vi "设置权限.vi"() -> (7 "Cancelled?":bool caption="取消？", 8 "验证成功":bool, 9 "权限选择 2":u16(ring) caption="确定" items=["Admin", "User"])   [LabVIEW 2017]
doc: "该模板用于创建能够进行事件处理的对话框。"
panel:
  in  "权限选择":u16(ring) caption="确定" items=["Admin", "User"]
  in  "修改密码":bool caption="确定"
  in  "密码":string
  in  "Cancel":bool caption="取消"
  in  "验证":bool caption="确定"
  # "权限验证"
  # "密码"
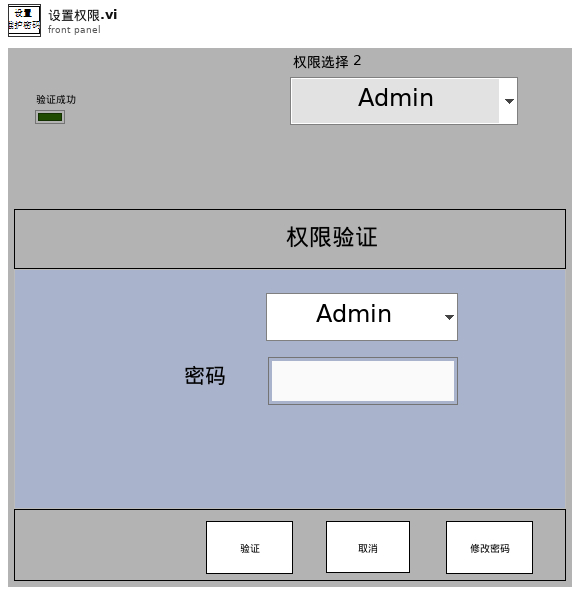
[diagram p1: front panel]
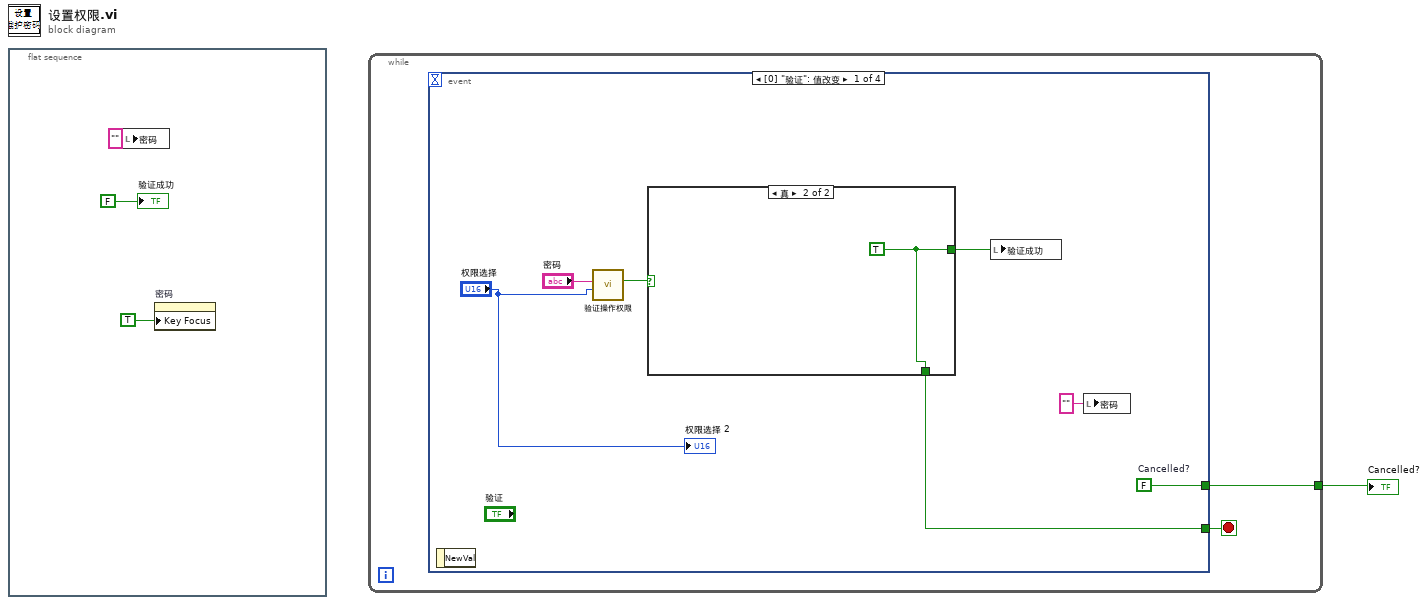
[diagram p0: block diagram]
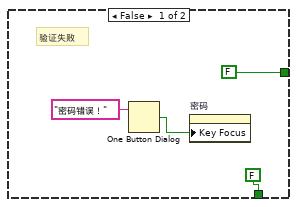
[diagram p2: hidden frame]
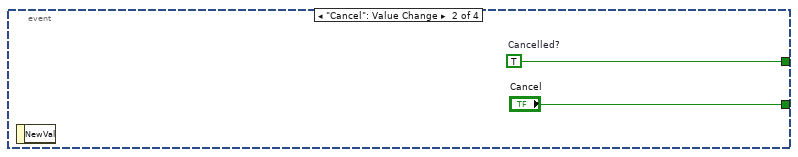
[diagram p3: hidden frame]
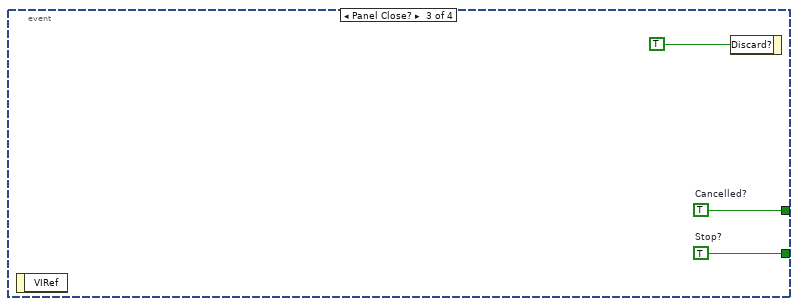
[diagram p4: hidden frame]
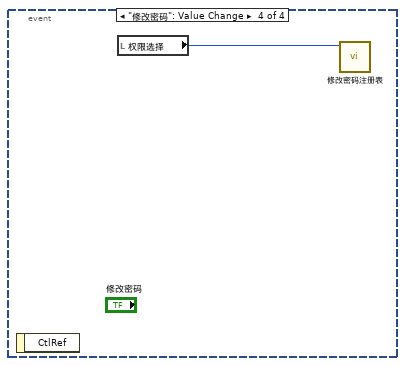
[diagram p5: hidden frame]
diagram:
  n1 = flat-sequence {
    frame #0 {
      n2 = local write "密码"("" ("用户名")) -> ()
      n3 = property on="密码" class="Str"("Key Focus"=TRUE ("键选中")) -> ()  [unwired: 2 in, 2 out]
      "验证成功" <- FALSE ("验证成功")
    }
  }
  n4 = while {
    tunnel: [w5] -> w1
    stop <- w6 stop-if-true
    n5 = event shown="[0] \"验证\": 值改变" {
      selector: _ -> [_ _ _ _]
      dyn-events: _ -> [_ _ _ _]
      timeout: _ -> [_ _ _ _]
      tunnel: [w8 "Cancel" w22 _] -> w6
      tunnel: [w13 w20 w21 _] -> w5
      event "验证": Value Change {
        w13 = FALSE  # Cancelled?
        n6 = event-data() -> ()  [unwired: 1 in, 1 out]
        n7 = call "验证操作权限.vi"("权限选择"="权限选择", "密码"="密码") -> ("验证成功"=w10:bool)  [unwired: 9 in]
        n8 = case shown="真" w10 {
          tunnel: [FALSE ("验证成功") w18] -> w9
          tunnel: [FALSE ("验证成功") w18] -> w8
          frame False {
            # "验证失败"
            n9 = One Button Dialog(message="密码错误！" ("消息")) -> (true=w14:bool)  [unwired: 1 in]
            n10 = property on="密码" class="Str"("Key Focus"=w14) -> ()  [unwired: 2 in, 2 out]
          }
          frame True {
            w18 = TRUE ("验证成功")
          }
        }
        n11 = local write "验证成功"(w9) -> ()
        n12 = local write "密码"("" ("用户名")) -> ()
        "权限选择 2" <- "权限选择"
      }
      event "Cancel": Value Change {
        w20 = TRUE  # Cancelled?
        n13 = event-data() -> ()  [unwired: 1 in, 1 out]
      }
      event Panel Close? {
        w21 = TRUE  # Cancelled?
        w22 = TRUE  # Stop?
        n14 = event-data() -> ()  [unwired: 1 in, 1 out]
        n15 = event-data("Discard?"=TRUE) -> ()  [unwired: 1 in, 1 out]
      }
      event "修改密码": Value Change {
        n16 = event-data() -> ()  [unwired: 1 in, 1 out]
        n17 = local read "权限选择"() -> (w24:u16)
        n18 = call "修改密码注册表.vi"("权限等级"=w24) -> ()  [unwired: 11 in]
      }
    }
  }
  "Cancelled?" <- w1
